vi "Measurement Logic.vi"() -> ()   [LabVIEW 2021, in "Dialog Box.lvlib"]
uses:
  Dialog Box.lvlib
  Measurement Configuration.ctl
  Array in.ctl
  Measurement Results.ctl
  <vilib>/MeasurementLink/MeasurementLink Measurement Server/Measure Call Context/Measure Call Context.lvclass
panel:
  out "measure call context out":refnum<class "Measure Call Context.lvclass">
  in  "measure call context in":refnum<class "Measure Call Context.lvclass">
  out "measurement results":T1
  in  "measurement configuration":T2
  out "error out":errorcluster
  in  "error in":errorcluster
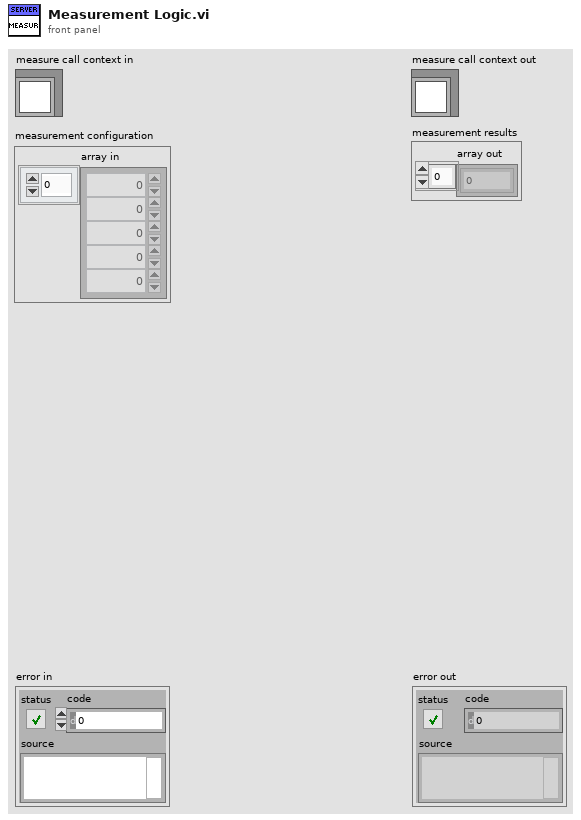
[diagram p1: front panel]
types:
  T1 = typedef "Dialog Box.lvlib/Measurement Results.ctl" = cluster{"array out":dbl[]}
  T2 = typedef "Dialog Box.lvlib/Measurement Configuration.ctl" = cluster{"array in":T3}
  T3 = typedef "Dialog Box.lvlib/Array in.ctl" = dbl[]
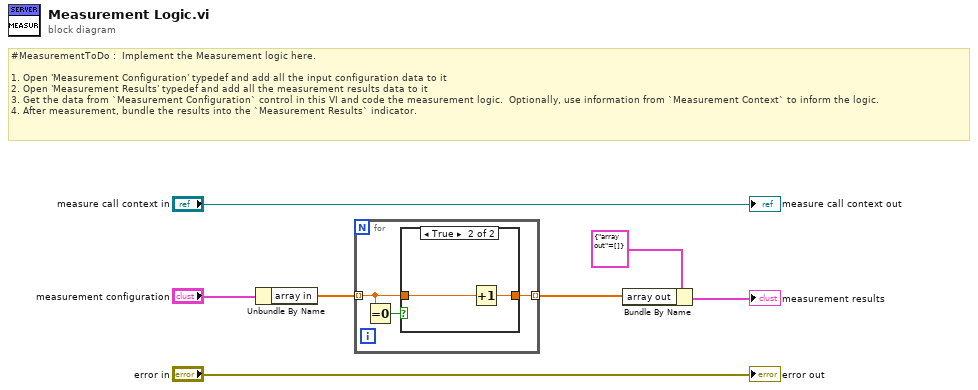
[diagram p0: block diagram]
diagram:
  # "#MeasurementToDo :  Implement the Measurement logic here.\n\n1. Open 'Measurement Configuration' typedef and add all the input configuration data to it\n2. Open 'Measurement Results' typedef and add all the measurement results data to it\n3. Get the data from `Measurement Configuration` control in this VI and code the measurement logic.  Optionally, use information from `Measurement Context` to inform the logic.\n4. After measurement, bundle the results into the `Measurement Results` indicator."
  n1 = Unbundle By Name("measurement configuration") -> ("array in"=w2:T3)
  n2 = for {
    tunnel: w2 -> [w9] mode=indexing
    tunnel: [w8] -> w1 mode=indexing
    n3 = Equal To 0?(x=w9) -> (x = 0?=w10:bool)
    n4 = case shown="True" w10 {
      tunnel: w9 -> [w11 w13]
      tunnel: [w11 w12] -> w8
      frame False {
      }
      frame True {
        n5 = Increment(x=w13) -> (x+1=w12:dbl)
      }
    }
  }
  n6 = Bundle By Name(cluster=T1 {"array out"=[]} ("Measurement Results"), "array out"=w1) -> (→"measurement results":T1)
  "error out" <- "error in"
  "measure call context out" <- "measure call context in"
